vi "Mean Freq Curves.vi"(11 "Set of Freq samples":T1) -> (0 "StdDev%":dbl, 3 "Mean Freq Curve":dbl[](array[numeric]))   [LabVIEW 2014]
uses:
  <vilib>/Analysis/Matrix/Datatypes/RealMatrix.ctl
  <vilib>/Analysis/NI_AALBase.lvlib
  <vilib>/Analysis/Matrix/NI_Matrix.lvlib
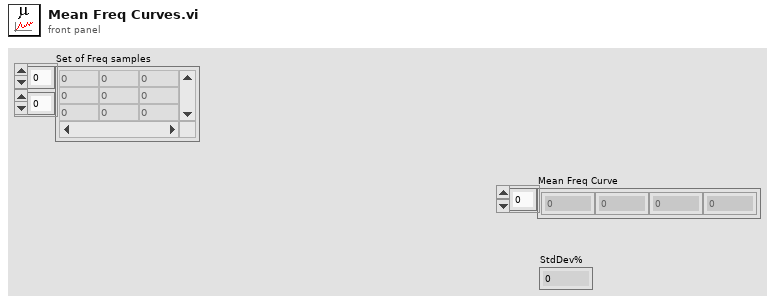
[diagram p1: front panel]
types:
  T1 = typedef "NI_Matrix.lvlib/RealMatrix.ctl" = dbl[][]
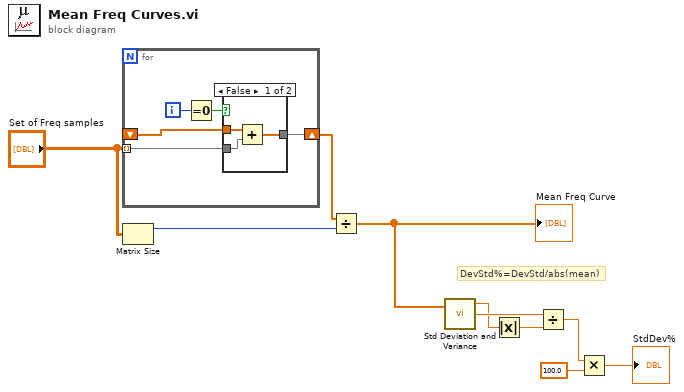
[diagram p0: block diagram]
diagram:
  # "DevStd%=DevStd/abs(mean)"
  n1 = for {
    tunnel: "Set of Freq samples" -> [w12] mode=indexing
    shift-right: [w13] -> w9
    shift-left: _ -> [w11]
    i -> [w15]
    n2 = Equal To 0?(x=w15) -> (x = 0?=w14:bool)
    n3 = case shown="False" w14 {
      tunnel: [w16 w19] -> w13
      tunnel: w12 -> [w17 w19]
      tunnel: w11 -> [w18 _]
      frame False {
        n4 = Add(x=w18, y=w17) -> (x+y=w16:dbl[])
      }
      frame True {
      }
    }
  }
  n5 = Matrix Size(0:"Set of Freq samples") -> (1:w10:i32)  [unwired: 1 out]
  n6 = Divide(x=w9, y=w10) -> (x/y=w7:dbl[])
  "Mean Freq Curve" <- w7
  n7 = call <vilib>:"Std Deviation and Variance.vi"("X"=w7) -> ("mean"=w4:dbl, "standard deviation"=w6:dbl)  [unwired: 1 in, 1 out]
  n8 = Absolute Value(x=w4) -> (abs(x)=w5:dbl)
  n9 = Divide(x=w6, y=w5) -> (x/y=w1:dbl)
  n10 = Multiply(x=w1, y=100.0) -> (x*y=→"StdDev%":dbl)
